vi "Global_OnCommand.vi"(10 "Command ID":string, 11 "Object":T1) -> ()   [LabVIEW 2020, in "Project Provider.lvlib"]
uses:
  Project Provider.lvlib
  <resource>/Framework/Providers/API/ItemRef.ctl
panel:
  out "error out":errorcluster
  in  "error in":errorcluster
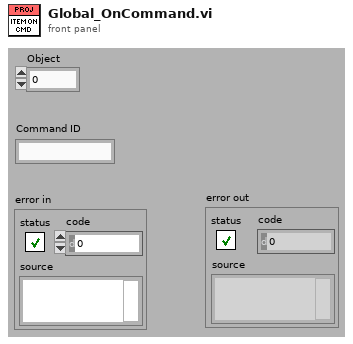
[diagram p1: front panel]
types:
  T1 = typedef "ItemRef.ctl" = u64
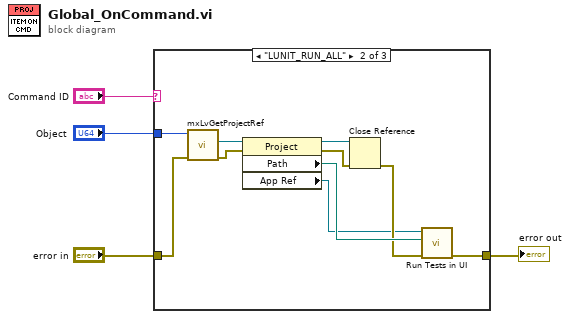
[diagram p0: block diagram]
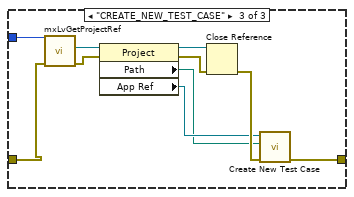
[diagram p3: hidden frame]
diagram:
  n1 = case shown="\"LUNIT_RUN_ALL\"" "Command ID" {
    tunnel: "error in" -> [w5 w10 w19]
    tunnel: [w5 w13 w25] -> w2
    tunnel: "Object" -> [_ w11 w20]
    frame Default {
    }
    frame "LUNIT_RUN_ALL" {
      n2 = call <resource>:"mxLvGetProjectRef.vi"("error in"=w10, "Item"=w11) -> ("error out"=w8:errorcluster, "Project Refnum"=w9:refnum<vi>)  [unwired: 7 in, 1 out]
      n3 = property class="Project"(reference=w9, error in=w8) -> (reference out=w14:refnum<vi>, error out=w15:errorcluster, "Path"=w12:path, "App Ref"=w6:refnum<vi>)
      n4 = Close Reference(reference=w14, error in (no error)=w15) -> (error out=w7:errorcluster)
      n5 = call "Run Tests in UI.vi"("error in (no error)"=w7, "Path"=w12, "Application"=w6) -> ("error out"=w13:errorcluster)  [unwired: 8 in]
    }
    frame "CREATE_NEW_TEST_CASE" {
      n6 = call <resource>:"mxLvGetProjectRef.vi"("error in"=w19, "Item"=w20) -> ("error out"=w21:errorcluster, "Project Refnum"=w22:refnum<vi>)  [unwired: 7 in, 1 out]
      n7 = property class="Project"(reference=w22, error in=w21) -> (reference out=w23:refnum<vi>, error out=w24:errorcluster, "Path"=w16:path, "App Ref"=w17:refnum<vi>)
      n8 = Close Reference(reference=w23, error in (no error)=w24) -> (error out=w18:errorcluster)
      n9 = call "Create New Test Case.vi"("error in (no error)"=w18, "Path"=w16, "Application"=w17) -> ("error out"=w25:errorcluster)  [unwired: 8 in]
    }
  }
  "error out" <- w2
